vi "Read ScalingData INI File.vi"(8 "error in":errorcluster, 11 "Path":path) -> (0 "error out":errorcluster, 3 "SmartRelay Scaling Cluster":T1)   [LabVIEW 2016]
uses:
  Controls/Smart Relay Scaling Cluster.ctl
  <vilib>/Utility/config.llb/Read Key (String).vi
  <vilib>/Utility/config.llb/NI_LVConfig.lvlib
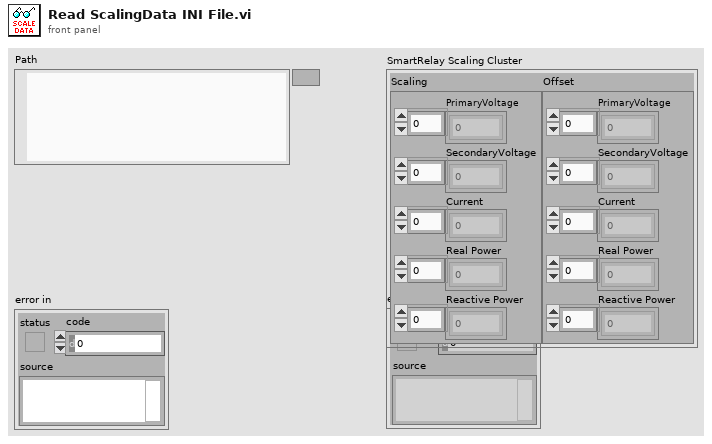
[diagram p1: front panel]
types:
  T1 = typedef "Smart Relay Scaling Cluster.ctl" = cluster{"Scaling":cluster{"PrimaryVoltage":dbl[], "SecondaryVoltage":dbl[], "Current":dbl[], "Real Power":dbl[], "Reactive Power":dbl[]}, "Offset":cluster{"PrimaryVoltage":dbl[], "SecondaryVoltage":dbl[], "Current":dbl[], "Real Power":dbl[], "Reactive Power":dbl[]}}
  T2 = typedef "NI_LVConfig.lvlib/Config Data RefNum.ctl" = refnum<k1>
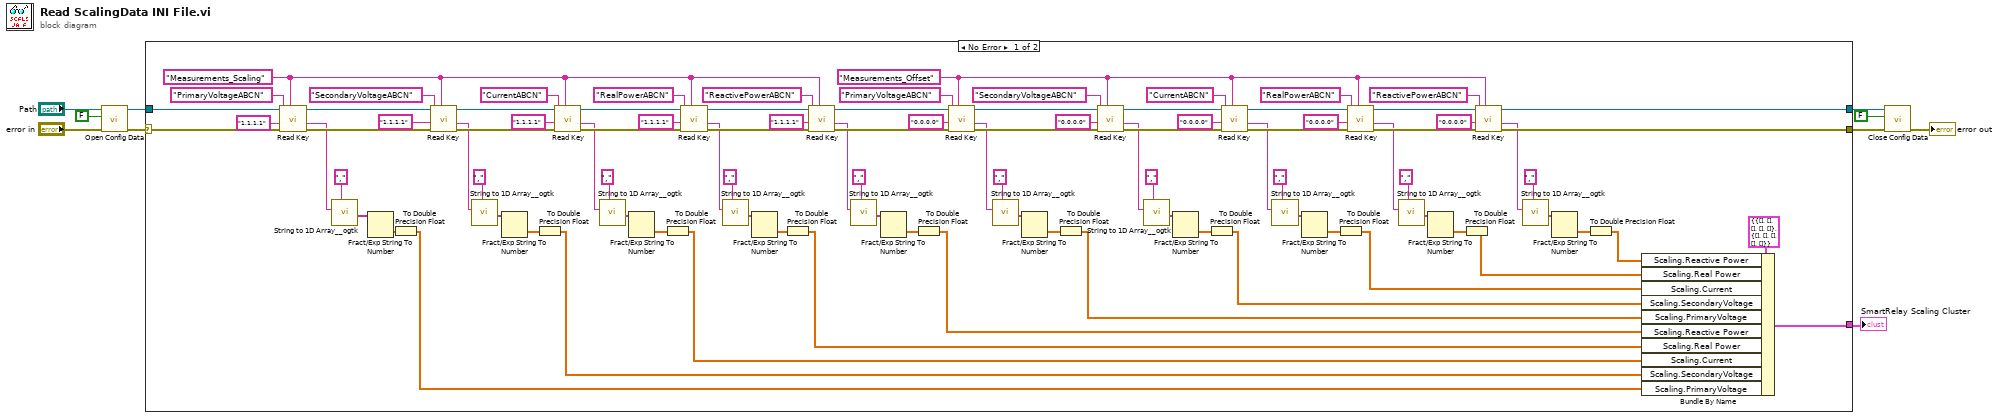
[diagram p0: block diagram]
diagram:
  n1 = call <vilib>:"Open Config Data.vi"("error in (no error)"="error in", "create file if necessary (T)"=FALSE, "configuration file path"="Path") -> ("error out"=w8:errorcluster, "refnum"=w7:T2)  [unwired: 6 in, 1 out]
  n2 = case shown="No Error" w8 {
    selector: w8 -> [w104 w107]
    tunnel: w7 -> [w105 w108]
    tunnel: [w71 w108] -> w6
    tunnel: [w72 w107] -> w5
    tunnel: [w103 _] -> w1
    frame No Error {
      w88 = "Measurements_Offset" ("section")
      w89 = "Measurements_Scaling" ("section")
      n3 = call-poly <vilib>:"Read Key.vi"("section"=w89, "error in (no error)"=w104, "default value"="1,1,1,1", "key"="PrimaryVoltageABCN", "refnum"=w105) -> ("error out"=w100:errorcluster, "value"=w69:string, "refnum out"=w99:T2)  [unwired: 3 in, 1 out]
      n4 = call <userlib>:"String to 1D Array__ogtk.vi"("delimiter (Tab)"=",", "string"=w69) -> ("Array of Strings"=w67:string[])  [unwired: 9 in]
      n5 = Fract/Exp String To Number(string=w67) -> (number=w66:dbl[])  [unwired: 3 in, 1 out]
      n6 = To Double Precision Float(number=w66) -> (double precision float=w65:dbl[])
      n7 = call-poly <vilib>:"Read Key.vi"("section"=w89, "error in (no error)"=w100, "default value"="1,1,1,1", "key"="SecondaryVoltageABCN", "refnum"=w99) -> ("error out"=w92:errorcluster, "value"=w37:string, "refnum out"=w95:T2)  [unwired: 3 in, 1 out]
      n8 = call <userlib>:"String to 1D Array__ogtk.vi"("delimiter (Tab)"=",", "string"=w37) -> ("Array of Strings"=w63:string[])  [unwired: 9 in]
      n9 = Fract/Exp String To Number(string=w63) -> (number=w64:dbl[])  [unwired: 3 in, 1 out]
      n10 = To Double Precision Float(number=w64) -> (double precision float=w28:dbl[])
      n11 = call-poly <vilib>:"Read Key.vi"("section"=w89, "error in (no error)"=w92, "default value"="1,1,1,1", "key"="CurrentABCN", "refnum"=w95) -> ("error out"=w91:errorcluster, "value"=w36:string, "refnum out"=w94:T2)  [unwired: 3 in, 1 out]
      n12 = call <userlib>:"String to 1D Array__ogtk.vi"("delimiter (Tab)"=",", "string"=w36) -> ("Array of Strings"=w60:string[])  [unwired: 9 in]
      n13 = Fract/Exp String To Number(string=w60) -> (number=w59:dbl[])  [unwired: 3 in, 1 out]
      n14 = To Double Precision Float(number=w59) -> (double precision float=w27:dbl[])
      n15 = call-poly <vilib>:"Read Key.vi"("section"=w89, "error in (no error)"=w91, "default value"="1,1,1,1", "key"="RealPowerABCN", "refnum"=w94) -> ("error out"=w90:errorcluster, "value"=w35:string, "refnum out"=w93:T2)  [unwired: 3 in, 1 out]
      n16 = call <userlib>:"String to 1D Array__ogtk.vi"("delimiter (Tab)"=",", "string"=w35) -> ("Array of Strings"=w57:string[])  [unwired: 9 in]
      n17 = Fract/Exp String To Number(string=w57) -> (number=w58:dbl[])  [unwired: 3 in, 1 out]
      n18 = To Double Precision Float(number=w58) -> (double precision float=w26:dbl[])
      n19 = call-poly <vilib>:"Read Key.vi"("section"=w89, "error in (no error)"=w90, "default value"="1,1,1,1", "key"="ReactivePowerABCN", "refnum"=w93) -> ("error out"=w73:errorcluster, "value"=w34:string, "refnum out"=w74:T2)  [unwired: 3 in, 1 out]
      n20 = call <userlib>:"String to 1D Array__ogtk.vi"("delimiter (Tab)"=",", "string"=w34) -> ("Array of Strings"=w54:string[])  [unwired: 9 in]
      n21 = Fract/Exp String To Number(string=w54) -> (number=w53:dbl[])  [unwired: 3 in, 1 out]
      n22 = To Double Precision Float(number=w53) -> (double precision float=w25:dbl[])
      n23 = call-poly <vilib>:"Read Key.vi"("section"=w88, "error in (no error)"=w73, "default value"="0,0,0,0", "key"="PrimaryVoltageABCN", "refnum"=w74) -> ("error out"=w77:errorcluster, "value"=w33:string, "refnum out"=w78:T2)  [unwired: 3 in, 1 out]
      n24 = call <userlib>:"String to 1D Array__ogtk.vi"("delimiter (Tab)"=",", "string"=w33) -> ("Array of Strings"=w51:string[])  [unwired: 9 in]
      n25 = Fract/Exp String To Number(string=w51) -> (number=w52:dbl[])  [unwired: 3 in, 1 out]
      n26 = To Double Precision Float(number=w52) -> (double precision float=w24:dbl[])
      n27 = call-poly <vilib>:"Read Key.vi"("section"=w88, "error in (no error)"=w77, "default value"="0,0,0,0", "key"="SecondaryVoltageABCN", "refnum"=w78) -> ("error out"=w85:errorcluster, "value"=w32:string, "refnum out"=w82:T2)  [unwired: 3 in, 1 out]
      n28 = call <userlib>:"String to 1D Array__ogtk.vi"("delimiter (Tab)"=",", "string"=w32) -> ("Array of Strings"=w48:string[])  [unwired: 9 in]
      n29 = Fract/Exp String To Number(string=w48) -> (number=w47:dbl[])  [unwired: 3 in, 1 out]
      n30 = To Double Precision Float(number=w47) -> (double precision float=w23:dbl[])
      n31 = call-poly <vilib>:"Read Key.vi"("section"=w88, "error in (no error)"=w85, "default value"="0,0,0,0", "key"="CurrentABCN", "refnum"=w82) -> ("error out"=w86:errorcluster, "value"=w31:string, "refnum out"=w83:T2)  [unwired: 3 in, 1 out]
      n32 = call <userlib>:"String to 1D Array__ogtk.vi"("delimiter (Tab)"=",", "string"=w31) -> ("Array of Strings"=w45:string[])  [unwired: 9 in]
      n33 = Fract/Exp String To Number(string=w45) -> (number=w46:dbl[])  [unwired: 3 in, 1 out]
      n34 = To Double Precision Float(number=w46) -> (double precision float=w22:dbl[])
      n35 = call-poly <vilib>:"Read Key.vi"("section"=w88, "error in (no error)"=w86, "default value"="0,0,0,0", "key"="RealPowerABCN", "refnum"=w83) -> ("error out"=w87:errorcluster, "value"=w30:string, "refnum out"=w84:T2)  [unwired: 3 in, 1 out]
      n36 = call <userlib>:"String to 1D Array__ogtk.vi"("delimiter (Tab)"=",", "string"=w30) -> ("Array of Strings"=w42:string[])  [unwired: 9 in]
      n37 = Fract/Exp String To Number(string=w42) -> (number=w41:dbl[])  [unwired: 3 in, 1 out]
      n38 = To Double Precision Float(number=w41) -> (double precision float=w21:dbl[])
      n39 = call-poly <vilib>:"Read Key.vi"("section"=w88, "error in (no error)"=w87, "default value"="0,0,0,0", "key"="ReactivePowerABCN", "refnum"=w84) -> ("error out"=w72:errorcluster, "value"=w29:string, "refnum out"=w71:T2)  [unwired: 3 in, 1 out]
      n40 = call <userlib>:"String to 1D Array__ogtk.vi"("delimiter (Tab)"=",", "string"=w29) -> ("Array of Strings"=w39:string[])  [unwired: 9 in]
      n41 = Fract/Exp String To Number(string=w39) -> (number=w40:dbl[])  [unwired: 3 in, 1 out]
      n42 = To Double Precision Float(number=w40) -> (double precision float=w20:dbl[])
      n43 = Bundle By Name(cluster=T1 {"Scaling"={"PrimaryVoltage"=[], "SecondaryVoltage"=[], "Current"=[], "Real Power"=[], "Reactive Power"=[]}, "Offset"={"PrimaryVoltage"=[], "SecondaryVoltage"=[], "Current"=[], "Real Power"=[], "Reactive Power"=[]}} ("SmartRelay Scaling Cluster"), "Scaling.Reactive Power"=w20, "Scaling.Real Power"=w21, "Scaling.Current"=w22, "Scaling.SecondaryVoltage"=w23, "Scaling.PrimaryVoltage"=w24, "Scaling.Reactive Power"=w25, "Scaling.Real Power"=w26, "Scaling.Current"=w27, "Scaling.SecondaryVoltage"=w28, "Scaling.PrimaryVoltage"=w65) -> (w103:T1)
    }
    frame Error {
    }
  }
  "SmartRelay Scaling Cluster" <- w1
  n44 = call <vilib>:"Close Config Data.vi"("error in (no error)"=w5, "write file if changed (T)"=FALSE, "refnum"=w6) -> ("error out"=→"error out":errorcluster)  [unwired: 7 in, 1 out]
